vi "Convert Transactions to String Arrays.vi"(8 "error in (no error)":errorcluster, 11 "Credit Statement in":refnum<class "Credit Statement.lvclass">) -> (0 "error out":errorcluster, 2 "String Arrays":string[](array[string]), 3 "Credit Statement out":refnum<class "Credit Statement.lvclass">)   [LabVIEW 2018, in "Credit Statement.lvclass"]
uses:
  Credit Statement.lvclass
  C:/GitRepos/Filthy-Lucre-Budgetizer/source/support/classes/Statement/Statement.lvclass
  Credit Record/Credit Transaction.lvclass
  Statement/Statement.lvclass
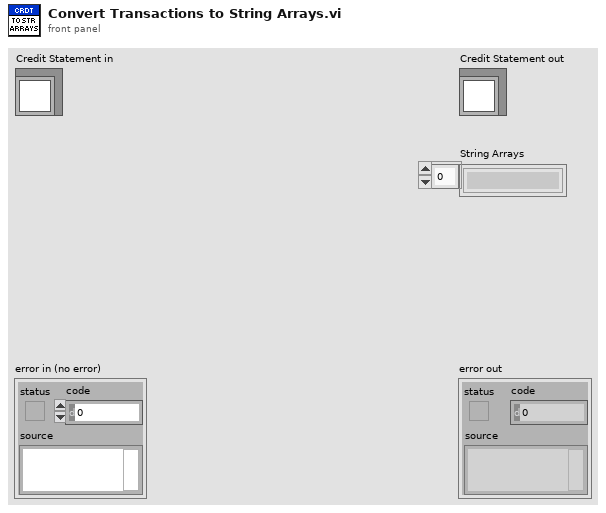
[diagram p1: front panel]
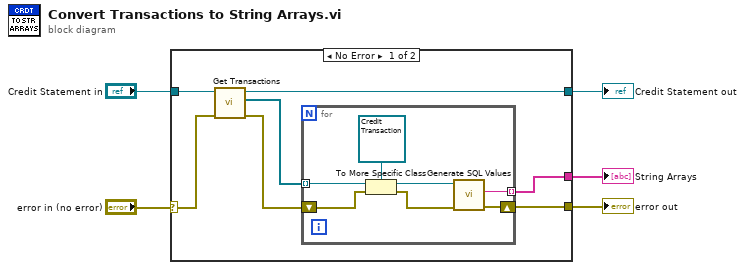
[diagram p0: block diagram]
diagram:
  n1 = case shown="No Error" "error in (no error)" {
    selector: "error in (no error)" -> [w8 w20]
    tunnel: "Credit Statement in" -> [w10 w21]
    tunnel: [w9 w21] -> w3
    tunnel: [w12 w20] -> w2
    tunnel: [w11 _] -> w1
    frame No Error {
      n2 = call "Get Transactions.vi"("error in (no error)"=w8, "Statement in"=w10) -> ("error out"=w7:errorcluster, "Transactions"=w6:refnum<class "Transaction.lvclass">[], "Statement out"=w9:refnum<class "Credit Statement.lvclass">)  [unwired: 7 in]
      n3 = for {
        tunnel: w6 -> [w17] mode=indexing
        shift-right: [w19] -> w12
        shift-left: w7 -> [w15]
        tunnel: [w18] -> w11 mode=indexing
        n4 = To More Specific Class(target class=refnum<class "Credit Transaction.lvclass"> refnum ("Credit Transaction.lvclass"), reference=w17, error in=w15) -> (specific class reference=w16:refnum<class "Credit Transaction.lvclass">, error out=w14:errorcluster)
        n5 = call-dynamic "Generate SQL Values.vi"("error in (no error)"=w14, "Credit Record in"=w16) -> ("error out"=w19:errorcluster, "SQL Values"=w18:string)  [unwired: 7 in, 1 out]
      }
    }
    frame Error {
    }
  }
  "error out" <- w2
  "Credit Statement out" <- w3
  "String Arrays" <- w1
